vi "OpenXL_Workbook.vi"(8 "error in":errorcluster, 10 "path":path, 11 "Refnum Cluster In":T1) -> (0 "error out":errorcluster, 3 "Refnum Cluster Out":T2)   [LabVIEW 2017, in "excel_configuration.lvlib"]
doc: "Opens the Excel workbook at path, prompting for a file when the path is empty, and adds the opened workbook reference to the reference cluster."
uses:
  excel_configuration.lvlib
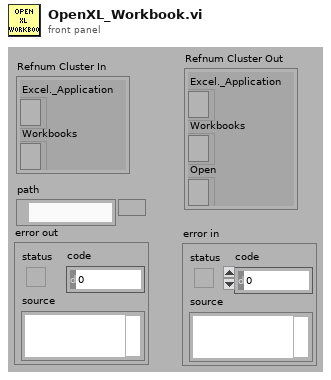
[diagram p1: front panel]
types:
  T1 = cluster{"Excel._Application":refnum<k7>, "Workbooks":refnum<k7>}
  T2 = cluster{"Excel._Application":refnum<k7>, "Workbooks":refnum<k7>, "Open":refnum<k7>}
  T3 = enum32{"existing file", "new file", "new or existing file", "existing dir", "new dir", "new or existing dir", "existing file (use LLBs)", "new file (use LLBs)", "new or existing file (use LLBs)", "new or existing file or directory (use LLBs)"}
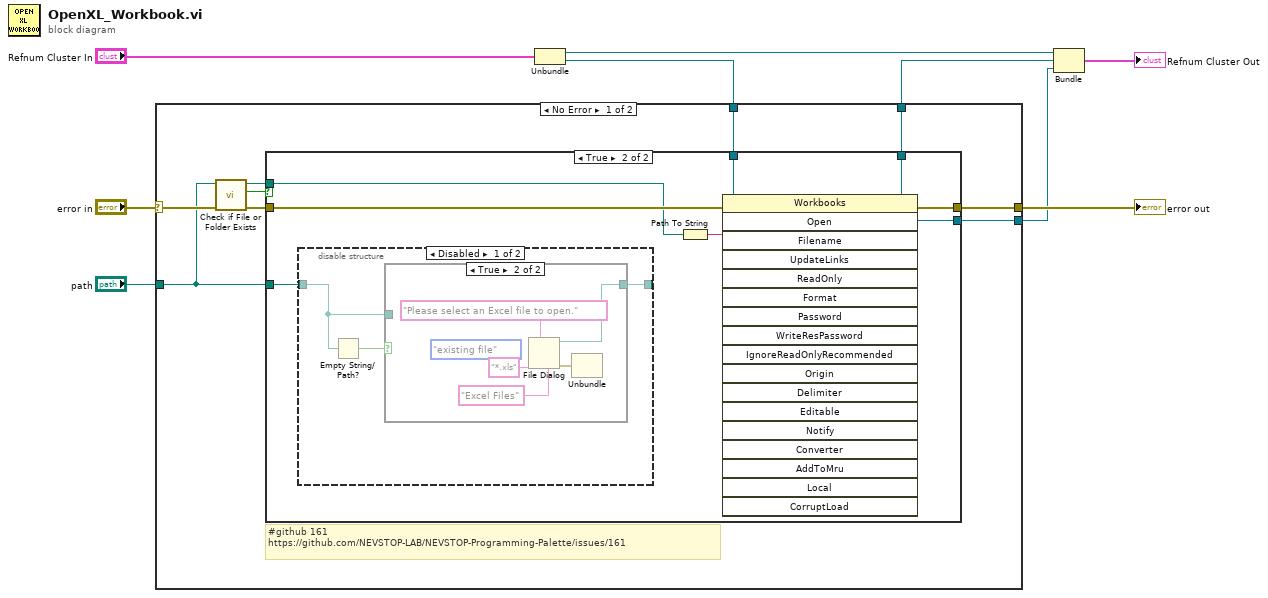
[diagram p0: block diagram]
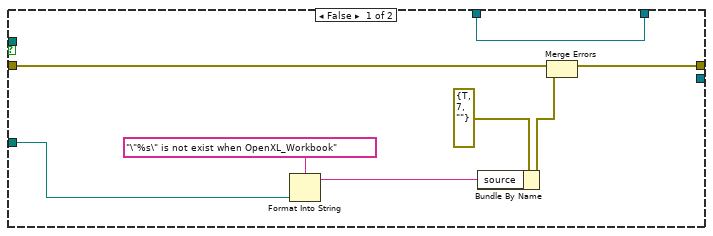
[diagram p2: hidden frame]
diagram:
  n1 = Unbundle("Refnum Cluster In") -> ("Excel._Application"=w2:refnum<k7>, "Workbooks"=w1:refnum<k7>)
  n2 = case shown="No Error" "error in" {
    selector: "error in" -> [w18 w46]
    tunnel: [w17 w46] -> w6
    tunnel: "path" -> [w16 _]
    tunnel: [w15 _] -> w4
    tunnel: [w14 w45] -> w3
    tunnel: w1 -> [w13 w45]
    frame No Error {
      # "#github 161\nhttps://github.com/NEVSTOP-LAB/NEVSTOP-Programming-Palette/issues/161"
      n3 = call <vilib>:"Check if File or Folder Exists.vi"("error in (no error)"=w18, "path"=w16) -> ("error out"=w12:errorcluster, "file or folder exists?"=w10:bool, "dup path"=w11:path)  [unwired: 7 in]
      n4 = case shown="True" w10 {
        tunnel: [w24 w34] -> w17
        tunnel: w16 -> [w20 w33]
        tunnel: [_ w32] -> w15
        tunnel: [w25 w31] -> w14
        tunnel: w13 -> [w25 w29]
        tunnel: w12 -> [w26 w28]
        tunnel: w11 -> [_ w27]
        frame False {
          n5 = Format Into String(format string="\"%s\" is not exist when OpenXL_Workbook", w20) -> (resulting string=w19:string)  [unwired: 2 in, 1 out]
          n6 = Bundle By Name(cluster=errorcluster {"status"=TRUE, "code"=7, "source"=""} ("error in"), "source"=w19) -> (w22:errorcluster)
          n7 = Merge Errors(w26, w22) -> (w24:errorcluster)
        }
        frame True {
          n8 = disable-structure shown="Disabled" {
            disable-tunnel: w33 -> [w36 w44]
            disable-tunnel: [w35 w44] -> _
            frame Disabled {
              n9 = Empty String/Path?(string/path=w36) -> (empty?=w37:bool)
              n10 = case shown="True" w37 {
                tunnel: w36 -> [w38 _]
                tunnel: [w38 w43] -> w35
                frame False {
                }
                frame True {
                  (unwired) T3."existing file" ("select mode (2)")
                  n11 = File Dialog(4:"Excel Files" ("pattern label"), 6:"*.xls" ("pattern"), 7:"Please select an Excel file to open." ("prompt")) -> (0:w39:errorcluster, 3:w43:path)  [unwired: 4 in, 2 out]
                  n12 = Unbundle(w39) -> ()  [unwired: 3 out]
                }
              }
            }
            frame Enabled {
            }
          }
          n13 = Path To String(path=w27) -> (string=w30:string)
          n14 = invoke on="Invoke Node" class="Workbooks" method="Open"(reference=w29, error in=w28, "Filename"=w30) -> (reference out=w31:refnum<k7>, error out=w34:errorcluster, "Open"=w32:refnum<k7>)  [unwired: 15 in, 15 out]
        }
      }
    }
    frame Error {
    }
  }
  "error out" <- w6
  n15 = Bundle("Excel._Application"=w2, "Workbooks"=w3, "Open"=w4) -> (→"Refnum Cluster Out":T2)  [unwired: 1 in]
